vi "Get Digits After Decimal.vi"(8 "error in (no error)":errorcluster, 11 "Numeric in":dbl) -> (0 "error out":errorcluster, 3 "Numeric out":i32)   [LabVIEW 2016]
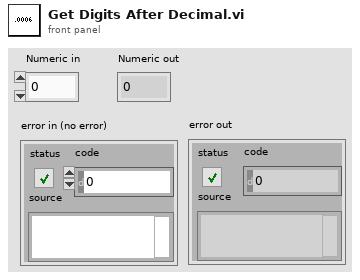
[diagram p1: front panel]
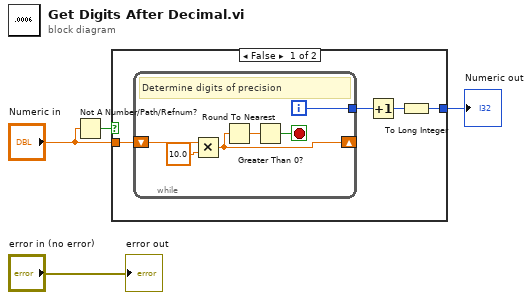
[diagram p0: block diagram]
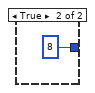
[diagram p2: hidden frame]
diagram:
  n1 = Not A Number/Path/Refnum?(number/path/refnum="Numeric in") -> (NaN/Path/Refnum?=w2:bool)
  n2 = case shown="False" w2 {
    tunnel: [w8 8] -> w4
    tunnel: "Numeric in" -> [w5 _]
    frame False {
      n3 = while {
        shift-right: [w9] -> _
        shift-left: w5 -> [w12]
        tunnel: [w13] -> w6
        i -> [w13]
        stop <- w14 stop-if-true
        # "Determine digits of precision"
        n4 = Multiply(x=w12, y=10.0 ("x")) -> (x*y=w9:dbl)
        n5 = Round To Nearest(number=w9) -> (nearest integer value=w10:dbl)
        n6 = Greater Than 0?(x=w10) -> (x > 0?=w14:bool)
      }
      n7 = Increment(x=w6) -> (x+1=w7:i32)
      n8 = To Long Integer(number=w7) -> (32bit integer=w8:i32)
    }
    frame True {
    }
  }
  "Numeric out" <- w4
  "error out" <- "error in (no error)"
